vi "Timing.vi"(10 "数组":u16[](array[numeric])) -> (1 "次数":i32[](array[numeric]), 2 "当前":u16, 3 "到":bool)   [LabVIEW 2020]
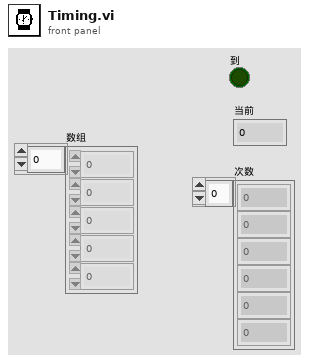
[diagram p1: front panel]
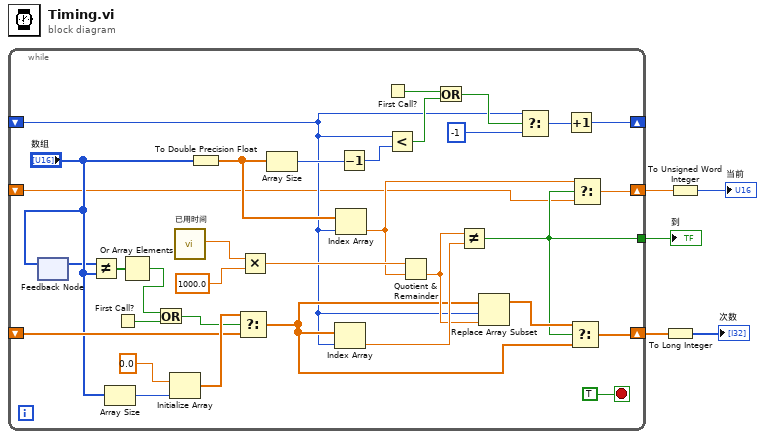
[diagram p0: block diagram]
diagram:
  n1 = while {
    shift-right: [w36] -> _
    shift-left: _ -> [w10]
    tunnel: [w9] -> w5
    shift-right: [w24] -> w3
    shift-left: _ -> [w19]
    shift-right: [w7] -> w1
    shift-left: _ -> [w6]
    stop <- TRUE stop-if-true
    n2 = feedback-in #1("数组") -> ()
    n3 = feedback #1() -> (w14:u16[])  [unwired: 1 in]
    n4 = Not Equal?(x=w14, y="数组") -> (x != y?=w13:bool[])
    n5 = Array Size(array="数组") -> (size(s)=w23:i32)
    n6 = First Call?() -> (First Call?: T/F=w17:bool)
    n7 = Or Array Elements(Boolean array=w13) -> (logical OR=w12:bool)
    n8 = Or(x=w12, y=w17) -> (x .or. y?=w16:bool)
    n9 = Initialize Array(0.0, w23) -> (w20:dbl[])
    n10 = call "已用时间"() -> ("Elapsed Time (s)"=w38:dbl)  [unwired: 12 in, 7 out]
    n11 = To Double Precision Float(number="数组") -> (double precision float=w21:dbl[])
    n12 = Select(t=w20, s=w16, f=w19) -> (s? t:f=w18:dbl[])
    n13 = Multiply(x=w38, y=1000.0) -> (x*y=w32:dbl)
    n14 = Array Size(array=w21) -> (size(s)=w35:i32)
    n15 = Index Array(array=w18, index=w10) -> (element=w31:dbl)
    n16 = Index Array(array=w21, index=w10) -> (element=w8:dbl)
    n17 = Decrement(x=w35) -> (x-1=w34:i32)
    n18 = First Call?() -> (First Call?: T/F=w28:bool)
    n19 = Less?(x=w10, y=w34) -> (x < y?=w29:bool)
    n20 = Quotient & Remainder(x=w32, y=w8) -> (floor(x/y)=w26:dbl)  [unwired: 1 out]
    n21 = Or(x=w28, y=w29) -> (x .or. y?=w27:bool)
    n22 = Not Equal?(x=w26, y=w31) -> (x != y?=w9:bool)
    n23 = Replace Array Subset(array=w18, new element=w26, index=w10) -> (w25:dbl[])
    n24 = Select(t=w10, s=w27, f=-1) -> (s? t:f=w33:i32)
    n25 = Increment(x=w33) -> (x+1=w36:i32)
    n26 = Select(t=w25, s=w9, f=w18) -> (s? t:f=w24:dbl[])
    n27 = Select(t=w8, s=w9, f=w6) -> (s? t:f=w7:dbl)
  }
  "到" <- w5
  n28 = To Long Integer(number=w3) -> (32bit integer=→"次数":i32[])
  n29 = To Unsigned Word Integer(number=w1) -> (unsigned 16bit integer=→"当前":u16)
